vi "PM100-Set Averaging.vi"(0 "VISA in":refnum<visa-resource-name>, 7 "Average time (ms)":dbl, 11 "error in (no error)":errorcluster) -> (4 "VISA out":refnum<visa-resource-name>, 15 "error out":errorcluster)   [LabVIEW 2015]
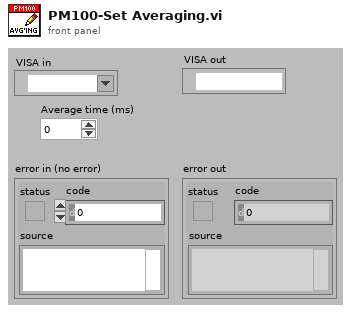
[diagram p1: front panel]
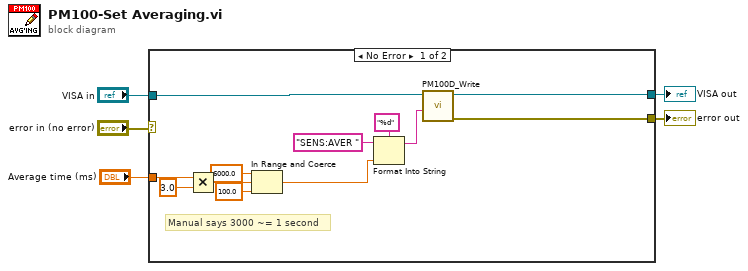
[diagram p0: block diagram]
diagram:
  n1 = case shown="No Error" "error in (no error)" {
    selector: "error in (no error)" -> [_ w19]
    tunnel: [w14 w19] -> w4
    tunnel: "VISA in" -> [w12 w18]
    tunnel: "Average time (ms)" -> [w11 _]
    tunnel: [w13 w18] -> w1
    frame No Error {
      # "Manual says 3000 ~= 1 second"
      n2 = Multiply(x=w11, y=3.0) -> (x*y=w9:dbl)
      n3 = In Range and Coerce(upper limit=6000.0, x=w9, lower limit=100.0) -> (coerced(x)=w8:dbl)  [unwired: 1 out]
      n4 = Format Into String(format string="%d", initial string="SENS:AVER " ("Command"), w8) -> (resulting string=w15:string)  [unwired: 1 in, 1 out]
      n5 = call "PM100D_Write.vi"("Command"=w15, "VISA in"=w12) -> ("error out"=w14:errorcluster, "VISA out"=w13:refnum<visa-resource-name>)  [unwired: 8 in]
    }
    frame Error {
    }
  }
  "error out" <- w4
  "VISA out" <- w1
